vi "Halvorsen_MEMP_Fast.vi"(0 "tolerance":dbl=1e-13, 1 "Error Analysis":u16(ring)=4 items=["Max", "Max_Norm", "Norm", "Last Value", "Last Constant"], 3 "Шаг h, с":dbl=0.001, 4 "k":i32=4, 5 "Время, с":dbl=30.0, 7 "Hmax":dbl=0.5, 8 "Parameter":dbl[](array[numeric])=[1.4, 1.4, 1.4], 10 "last_point_Thomas":dbl[](array[numeric])=[2.3727475682665875, 0.23609824454436878, 0.4447912442126299], 13 "Hmin":dbl=0.001, 15 "Points count":i32=2, 18 "n":i32[](array[numeric])=[2, 4, 6, 8, 10, 12, 14, 16, 18, 20, 22], 19 "Ext.Type":u16(ring) items=["FNode", "MathScript", "ECD8 Arrays", "ECD8 Fnode", "ECD8 FnodeDiv", "FNode Exp"]) -> (6 "Elapsed Time":dbl=0.013410782656137599, 12 "Number of steps":i32=365, 14 "Error Estimation":dbl=1.511027811908779e-13, 17 "Rejected steps":i32=1)   [LabVIEW 2016]
uses:
  <vilib>/Analysis/_algsub.llb/Real Vector Norm.vi
  <vilib>/Analysis/5stat.llb/RMS (DBL).vi
  <vilib>/Analysis/NI_AALBase.lvlib
  <vilib>/Analysis/NI_AALPro.lvlib
panel:
  in  "Initial Conditions":dbl[](array[numeric])=[1.0, 0.0, 1.0]
  out "Last Value Reference":dbl[](array[numeric])=[2.372747575181197, 0.2360982473599586, 0.44479123807251236] format="%#_15f"
  out "Rejected Steps":i32[](graph)=[0, 1, 0, 0, 0, 0, 0, 0, 0, 0, 0, 0, 0, 0, 0, 0, 0, 0, 0, 0, 0, 0, 0, 0, 0, 0, 0, 0, 0, 0, 0, 0, 0, 0, 0, 0, 0, 0, 0, 0, 0, 0, 0, 0, 0, 0, 0, 0, 0, 0, 0, 0, 0, 0, 0, 0, 0, 0, 0, 0, 0, 0, 0, 0, 0, 0, 0, 0, 0, 0, 0, 0, 0, 0, 0, 0, 0, 0, 0, 0, 0, 0, 0, 0, 0, 0, 0, 0, 0, 0, 0, 0, 0, 0, 0, 0, 0, 0, 0, 0, 0, 0, 0, 0, 0, 0, 0, 0, 0, 0, 0, 0, 0, 0, 0, 0, 0, 0, 0, 0, 0, 0, 0, 0, 0, 0, 0, 0, 0, 0, 0, 0, 0, 0, 0, 0, 0, 0, 0, 0, 0, 0, 0, 0, 0, 0, 0, 0, 0, 0, 0, 0, 0, 0, 0, 0, 0, 0, 0, 0, 0, 0, 0, 0, 0, 0, 0, 0, 0, 0, 0, 0, 0, 0, 0, 0, 0, 0, 0, 0, 0, 0, 0, 0, 0, 0, 0, 0, 0, 0, 0, 0, 0, 0, 0, 0, 0, 0, 0, 0, 0, 0, 0, 0, 0, 0, 0, 0, 0, 0, 0, 0, 0, 0, 0, 0, 0, 0, 0, 0, 0, 0, 0, 0, 0, 0, 0, 0, 0, 0, 0, 0, 0, 0, 0, 0, 0, 0, 0, 0, 0, 0, 0, 0, 0, 0, 0, 0, 0, 0, 0, 0, 0, 0, 0, 0, 0, 0, 0, 0, 0, 0, 0, 0, 0, 0, 0, 0, 0, 0, 0, 0, 0, 0, 0, 0, 0, 0, 0, 0, 0, 0, 0, 0, 0, 0, 0, 0, 0, 0, 0, 0, 0, 0, 0, 0, 0, 0, 0, 0, 0, 0, 0, 0, 0, 0, 0, 0, 0, 0, 0, 0, 0, 0, 0, 0, 0, 0, 0, 0, 0, 0, 0, 0, 0, 0, 0, 0, 0, 0, 0, 0, 0, 0, 0, 0, 0, 0, 0, 0, 0, 0, 0, 0, 0, 0, 0, 0, 0, 0, 0, 0, 0, 0, 0, 0, 0, 0, 0, 0, 0, 0, 0, 0, 0, 0]
  out "Last Value":dbl[](array[numeric])=[2.372747568266689, 0.23609824454439432, 0.4447912442125211] format="%#_15f"
  out "Step time variation":dbl[](graph)=[0.011369601445039734, 0.015451963867235463]
  out "Real Error":dbl[][](graph)=[[0.0, 0.0, 0.0], [-3.3306690738754696e-16, 1.3010426069826053e-18, -2.220446049250313e-16], [2.269606724780715e-11, 7.413888947205294e-12, 4.742872761198669e-13], [4.520905871885361e-11, 1.3305856416678807e-11, 1.909139513145419e-12], [7.047429306794584e-11, 1.876210298235037e-11, 4.3729464493935666e-12], [9.8196561992836e-11, 2.377908980832899e-11, 8.00870481043603e-12], [1.2789103109867028e-10, 2.8306301746994222e-11, 1.2933210058463374e-11], [1.5886247872742842e-10, 3.224581712757413e-11, 1.921751646705161e-11], [1.901305779483664e-10, 3.5431102496374933e-11, 2.6864288571459838e-11], [2.2054869042165137e-10, 3.7660319307519785e-11, 3.5733416225980363e-11], [2.49152254383489e-10, 3.872691056727717e-11, 4.555289478958002e-11], [2.7525737245071014e-10, 3.842048901248063e-11, 5.593414620364001e-11], [2.9841329407531703e-10, 3.652400604181594e-11, 6.640399341506509e-11], [3.1840730052579147e-10, 3.281785954101224e-11, 7.643041755045488e-11], [3.351821042940628e-10, 2.706557200582438e-11, 8.546230390038545e-11], [3.488276334451257e-10, 1.9006352047767905e-11, 9.29043508790528e-11], [3.5940028730863105e-10, 8.411493723770036e-12, 9.811396139980388e-11], [3.670319603799044e-10, -4.916067553040193e-12, 1.003956917600135e-10], [3.719102803501073e-10, -2.1124657578752704e-11, 9.899281394609716e-11], [3.7423997234498074e-10, -4.012123966390391e-11, 9.306999615432687e-11], [3.7433145472220986e-10, -6.147837794401312e-11, 8.178391297519738e-11], [3.725815211907957e-10, -8.384315464127212e-11, 6.466382984626762e-11], [3.6960612348480026e-10, -1.0517831050549376e-10, 4.1951775386905865e-11], [3.6611647047379847e-10, -1.2337975086040842e-10, 1.4587886454364707e-11], [3.626872135953363e-10, -1.37165390157179e-10, -1.645572567099407e-11], [3.5965053157838156e-10, -1.458719811608944e-10, -5.041966844032686e-11], [3.571414275427287e-10, -1.493618562165011e-10, -8.721334765482425e-11], [3.5512126572712077e-10, -1.473818844743846e-10, -1.2639578272910512e-10], [3.535016723787976e-10, -1.398532400997965e-10, -1.6765255850259564e-10], [3.521241076498427e-10, -1.2682921379791878e-10, -2.1040236219960207e-10], [3.508104917671062e-10, -1.0861400667749876e-10, -2.537507981514864e-10], [3.493663136566738e-10, -8.573142196155459e-11, -2.969247070438996e-10], [3.4760949674250696e-10, -5.873412867174466e-11, -3.3953106992612447e-10], [3.453877184256271e-10, -2.8161695198036796e-11, -3.812243853928976e-10], [3.4256997238912845e-10, 5.6277205118249185e-12, -4.2203796013495776e-10], [3.3902347595926585e-10, 4.23832080542752e-11, -4.6196557690336704e-10], [3.346389831904162e-10, 8.190870204316525e-11, -5.009663794908192e-10], [3.2927260917858803e-10, 1.241433622567456e-10, -5.391123103493101e-10], [3.22812887532109e-10, 1.689934858717379e-10, -5.762417210064541e-10], [3.150950611541248e-10, 2.1638091318720853e-10, -6.122209406100865e-10], [3.0594549116358394e-10, 2.664068965430033e-10, -6.470637359257125e-10], [2.951319189037349e-10, 3.190443464973214e-10, -6.805551677757649e-10], [2.823865585810381e-10, 3.74259956359424e-10, -7.124398848645797e-10], [2.673807841802045e-10, 4.321243363136773e-10, -7.425686732176473e-10], [2.497113626986902e-10, 4.924811669582141e-10, -7.705183158179807e-10], [2.2885560113650172e-10, 5.552565074395943e-10, -7.960032633036462e-10], [2.0431967229228576e-10, 6.199005753160236e-10, -8.183853594800894e-10], [1.7554580011847065e-10, 6.856524237264239e-10, -8.370841797500361e-10], [1.421134321333284e-10, 7.512155342226379e-10, -8.514549065807842e-10], [1.0379430648299603e-10, 8.149392272116529e-10, -8.609801760428581e-10], [6.043654465770487e-11, 8.754437175184648e-10, -8.655169914106864e-10], [1.1836309710133719e-11, 9.318430471694228e-10, -8.651319660657464e-10], [-4.217692861629985e-11, 9.834488778892592e-10, -8.599161382960574e-10], [-1.0181278042864506e-10, 1.0298446539991346e-09, -8.499481118917629e-10], [-1.6732792929019524e-10, 1.070767030597608e-09, -8.352358804586402e-10], [-2.389262121482716e-10, 1.1059779758681998e-09, -8.157035047418049e-10], [-3.1656099963583983e-10, 1.1351612982934967e-09, -7.912341892790664e-10], [-4.003752884784717e-10, 1.1581864356458027e-09, -7.615919006553895e-10], [-4.902416250729402e-10, 1.1748908512743128e-09, -7.264904233750258e-10], [-5.856382045976716e-10, 1.1851151171526908e-09, -6.856295531321166e-10], [-6.8566397004588e-10, 1.1888712236896026e-09, -6.387324003043204e-10], [-7.88806797658026e-10, 1.1863856563820718e-09, -5.856388707314863e-10], [-8.927312222795081e-10, 1.1783156672606765e-09, -5.264999547449634e-10], [-9.954423951796798e-10, 1.1657244058937977e-09, -4.614766346833221e-10], [-1.095240786952445e-09, 1.1499659002822682e-09, -3.908151580134245e-10], [-1.1909015995570371e-09, 1.1324967630343963e-09, -3.1480018591878434e-10], [-1.282120631884709e-09, 1.1146310541221283e-09, -2.334257231950687e-10], [-1.3687890820790471e-09, 1.0976135556006739e-09, -1.4672596471143606e-10], [-1.4512280266387734e-09, 1.0825158547334013e-09, -5.4545479244438866e-11], [-1.5297518807244614e-09, 1.0703331554395845e-09, 4.319211655001709e-11], [-1.6049179762944732e-09, 1.0619474188899858e-09, 1.467421739675956e-10], [-1.6772010447141383e-09, 1.0581988618696414e-09, 2.5620083832222917e-10], [-1.7472245872340864e-09, 1.0598388833216177e-09, 3.718001462260645e-10], [-1.8155201786385078e-09, 1.0675997863529574e-09, 4.936342445915898e-10], [-1.8827255310327473e-09, 1.082119727158215e-09, 6.218509041033826e-10], [-1.9495254299783937e-09, 1.1040359737535255e-09, 7.567088067261807e-10], [-2.0165042968756097e-09, 1.1339031935619914e-09, 8.982441457305868e-10], [-2.0842634285145323e-09, 1.1722054438223495e-09, 1.0464090705042395e-09], [-2.153461409193369e-09, 1.219389034190499e-09, 1.20131138370283e-09], [-2.224737727374304e-09, 1.2758190059969365e-09, 1.3629377626500627e-09], [-2.298704337988511e-09, 1.3418079980453967e-09, 1.5312439094472552e-09], [-2.375939889276424e-09, 1.4175438600716461e-09, 1.706089047814885e-09], [-2.457072767469981e-09, 1.503223767684858e-09, 1.887440093106818e-09], [-2.542607457911572e-09, 1.5988392831900455e-09, 2.074995175682659e-09], [-2.633085305348004e-09, 1.7043637612346174e-09, 2.2685439082792414e-09], [-2.7290245618871722e-09, 1.8196844031592718e-09, 2.467889892443509e-09], [-2.8308635435791984e-09, 1.944516547780495e-09, 2.6726565405255087e-09], [-2.9390800904138814e-09, 2.0785546617219097e-09, 2.882632688105957e-09], [-3.0538354067743967e-09, 2.221035355631784e-09, 3.0969237174716113e-09], [-3.175532725663288e-09, 2.3713093710853173e-09, 3.315203667142441e-09], [-3.3041729352589755e-09, 2.5281736704130253e-09, 3.5363526551535074e-09], [-3.4395992720703816e-09, 2.690032196994707e-09, 3.7589874546384294e-09], [-3.581490215509575e-09, 2.8548599040334466e-09, 3.981411866860185e-09], [-3.729302644472909e-09, 3.020099725858927e-09, 4.201519576696455e-09], [-3.882181243142213e-09, 3.1824853863327007e-09, 4.41654868232888e-09], [-4.03904820700518e-09, 3.3380214148337473e-09, 4.62318183735988e-09], [-4.199012693106852e-09, 3.4821168171106365e-09, 4.8179054079611205e-09], [-4.36111946555684e-09, 3.608756848905159e-09, 4.995886815351014e-09], [-4.523064811579047e-09, 3.708372275923466e-09, 5.1477349050088606e-09], [-4.665753783328341e-09, 3.761142508551529e-09, 5.241526990218404e-09], [-4.778935247529148e-09, 3.7647316375455375e-09, 5.27045962428474e-09], [-4.867581893108763e-09, 3.7267104957550146e-09, 5.2449036225254986e-09], [-4.934693764724329e-09, 3.651821955941159e-09, 5.168978356451248e-09], [-4.982243506646e-09, 3.5434499778830286e-09, 5.043296669171582e-09], [-5.011369763607831e-09, 3.4055585018677448e-09, 4.867777292361097e-09], [-5.0233026627211075e-09, 3.2424267715214228e-09, 4.641494300017257e-09], [-5.019344051504504e-09, 3.0601361444837494e-09, 4.3650949521634175e-09], [-5.001047020947169e-09, 2.8651285788328096e-09, 4.0389944722107884e-09], [-4.970253653091561e-09, 2.6656907792244056e-09, 3.6668996727939884e-09], [-4.928755514832517e-09, 2.4691173550195344e-09, 3.250662405918092e-09], [-4.877563686278563e-09, 2.2806920796369923e-09, 2.784903418984186e-09], [-4.8176391764798154e-09, 2.1081003609424442e-09, 2.268234933211488e-09], [-4.749119153490966e-09, 1.9586847699315513e-09, 1.6932069080155543e-09], [-4.6732550607053724e-09, 1.8433663484529461e-09, 1.0728617994004708e-09], [-4.593981389744428e-09, 1.7714603117724437e-09, 4.6040993240126227e-10], [-4.512853715721299e-09, 1.7417605135960912e-09, -1.2046008635024918e-10], [-4.429691658619506e-09, 1.749222100499992e-09, -6.649663042423981e-10], [-4.344329868066765e-09, 1.787636705330442e-09, -1.1674967659303093e-09], [-4.256868690877269e-09, 1.849461916947348e-09, -1.622452394656193e-09], [-4.166818112771864e-09, 1.927224602127353e-09, -2.0314718796043962e-09], [-4.073079096222898e-09, 2.0147226109656913e-09, -2.40032660414613e-09], [-3.97467686541475e-09, 2.1065007516085643e-09, -2.733283821498844e-09], [-3.8703744653645344e-09, 2.198025761401823e-09, -3.0349061042045378e-09], [-3.759503153233368e-09, 2.2845947356131546e-09, -3.307053519918668e-09], [-3.6415166437819835e-09, 2.3617054978331e-09, -3.551469340834501e-09], [-3.515302271495102e-09, 2.4255042418985795e-09, -3.771099210680973e-09], [-3.3810777511078527e-09, 2.471259641367851e-09, -3.966069916927495e-09], [-3.2386722192967454e-09, 2.4946693599758873e-09, -4.137856501884585e-09], [-3.088418742969168e-09, 2.4911006590855322e-09, -4.287481480957922e-09], [-2.93190971500934e-09, 2.4558959310638784e-09, -4.415178667116493e-09], [-2.7711624106530053e-09, 2.3847972485668834e-09, -4.521777174915087e-09], [-2.608735893971925e-09, 2.2737820515317253e-09, -4.608395665073317e-09], [-2.4485620198078095e-09, 2.1201280731020233e-09, -4.676016907012581e-09], [-2.2952866274295047e-09, 1.922894732331315e-09, -4.725975166763874e-09], [-2.152907629948686e-09, 1.6809034164566583e-09, -4.760234872946967e-09], [-2.026153245182627e-09, 1.3948939781016634e-09, -4.780551510208397e-09], [-1.9199142275994063e-09, 1.0684315654430065e-09, -4.7886514753514575e-09], [-1.8381887123553042e-09, 7.05777658538409e-10, -4.786272822521198e-09], [-1.7843810873330312e-09, 3.1537883415921897e-10, -4.774996509304685e-09], [-1.7602175272912746e-09, -9.689493651876546e-11, -4.756135596473143e-09], [-1.766607971021017e-09, -5.262750235601743e-10, -4.73051503524502e-09], [-1.8039589821938762e-09, -9.692806557382028e-10, -4.698394673319228e-09], [-1.8729175987886038e-09, -1.4267333980910735e-09, -4.659212571311855e-09], [-1.9751693614011856e-09, -1.902701107781013e-09, -4.611367121487575e-09], [-2.112907848683676e-09, -2.39911290833561e-09, -4.55224062612114e-09], [-2.280200916970898e-09, -2.8884983294119593e-09, -4.480942660325948e-09], [-2.456705505693435e-09, -3.321690478230721e-09, -4.401077169369216e-09], [-2.632064344254559e-09, -3.7018246246134368e-09, -4.312903090220033e-09], [-2.8018853903688523e-09, -4.040882295441861e-09, -4.21502360792303e-09], [-2.9626983089059422e-09, -4.3464973842333166e-09, -4.105980500046513e-09], [-3.1108005060787036e-09, -4.622784821606274e-09, -3.984646002042069e-09], [-3.2425311324857375e-09, -4.87253881686911e-09, -3.85004728098437e-09], [-3.3539198085463795e-09, -5.0973394394304705e-09, -3.7016664178324277e-09], [-3.441230411738161e-09, -5.298790739516335e-09, -3.5389657870865676e-09], [-3.5004914522573927e-09, -5.4782338665404495e-09, -3.3616257555380002e-09], [-3.5272615939163643e-09, -5.636151101384712e-09, -3.1703967229290697e-09], [-3.5172265100413824e-09, -5.7729803160100346e-09, -2.966862755471311e-09], [-3.4662375192340278e-09, -5.889586596197205e-09, -2.7529919455204777e-09], [-3.3704501412046284e-09, -5.9867684143455335e-09, -2.5318758201109404e-09], [-3.2270670580203387e-09, -6.065342006422725e-09, -2.30813290702514e-09], [-3.034582807259767e-09, -6.126536611361644e-09, -2.0870680739193403e-09], [-2.7925790568872344e-09, -6.171990030168217e-09, -1.874124300194069e-09], [-2.5033464190471477e-09, -6.203366709200964e-09, -1.6756662724048965e-09], [-2.1715211850903415e-09, -6.222673043509985e-09, -1.4976326845328458e-09], [-1.8041537153123954e-09, -6.232016236396021e-09, -1.3450718316931898e-09], [-1.4073324727803538e-09, -6.233577209968644e-09, -1.2209957489517365e-09], [-9.88697568260477e-10, -6.2293068481267255e-09, -1.1275709255187394e-09], [-5.555640392174155e-10, -6.221014370311195e-09, -1.0656620030857766e-09], [-1.1039880121188617e-10, -6.210144842810905e-09, -1.0349947565657658e-09], [3.416795735233791e-10, -6.1979439358594846e-09, -1.0353415902386587e-09], [7.983995686799972e-10, -6.185412182446726e-09, -1.0661789229260421e-09], [1.2571450547227414e-09, -6.17340312203396e-09, -1.1269785105127994e-09], [1.7155787901401709e-09, -6.162597099290679e-09, -1.2171479379929906e-09], [2.1712422970665557e-09, -6.153543008480256e-09, -1.3359688910696832e-09], [2.622194905654851e-09, -6.146612108182126e-09, -1.4826724292760218e-09], [3.0670750383876566e-09, -6.1420393215882996e-09, -1.6565446792071725e-09], [3.50443807306533e-09, -6.139857955389516e-09, -1.8567787307688377e-09], [3.93260091158254e-09, -6.139864616727664e-09, -2.0823258672919565e-09], [4.3493675327965775e-09, -6.141575248364006e-09, -2.3316473196643983e-09], [4.752593429913077e-09, -6.144155406673235e-09, -2.602883242275311e-09], [5.139857428559935e-09, -6.146263498152393e-09, -2.893587813801446e-09], [5.507105438340432e-09, -6.145950859348659e-09, -3.199704945444637e-09], [5.847144546322625e-09, -6.140574271285004e-09, -3.513682456102174e-09], [6.151850584501517e-09, -6.126912754922387e-09, -3.825169070381662e-09], [6.414956121858495e-09, -6.101413152492796e-09, -4.123291486024527e-09], [6.631765803177814e-09, -6.0605684915060465e-09, -4.397124664379248e-09], [6.800017438024497e-09, -6.0011866587217355e-09, -4.637271011631583e-09], [6.919676831529387e-09, -5.920428147732082e-09, -4.836907985250605e-09], [6.991337953010657e-09, -5.816171100292422e-09, -4.99025554212551e-09], [7.016646819124617e-09, -5.686787929448656e-09, -5.093523824939439e-09], [6.997607382430715e-09, -5.5315445557369e-09, -5.143962145126579e-09], [6.93653423589069e-09, -5.34997135481774e-09, -5.14003661855611e-09], [6.835543020500268e-09, -5.141924219742577e-09, -5.080567078152853e-09], [6.695762388986282e-09, -4.906637540713632e-09, -4.96370322622397e-09], [6.517690831486789e-09, -4.643849527141697e-09, -4.786623541974677e-09], [6.3030773933547835e-09, -4.3561028117977685e-09, -4.547633380980187e-09], [6.062590429678494e-09, -4.0566199288605276e-09, -4.256597740948109e-09], [5.81213410733028e-09, -3.762749001268162e-09, -3.9333607482205935e-09], [5.556922699767597e-09, -3.4795997194692063e-09, -3.586301033919881e-09], [5.295042071473688e-09, -3.206297449764861e-09, -3.2140152761428453e-09], [5.029283212110158e-09, -2.9478257612680636e-09, -2.8218201109098118e-09], [4.780692619554827e-09, -2.7233629795730963e-09, -2.4437900592033657e-09], [4.5569121809307944e-09, -2.537292265181179e-09, -2.095620121878028e-09], [4.351461524443323e-09, -2.382397723543761e-09, -1.7708918775838356e-09], [4.159282807059128e-09, -2.2535548982460796e-09, -1.4644823131959583e-09], [3.97693200593352e-09, -2.147515165695779e-09, -1.1733036764383087e-09], [3.801982451090424e-09, -2.062131465585537e-09, -8.956360098011373e-10], [3.6326260888230877e-09, -1.9958757424554108e-09, -6.305684863150418e-10], [3.467354514619103e-09, -1.947516592437637e-09, -3.776414736478273e-10], [3.304651441382589e-09, -1.9159627218101605e-09, -1.3632250883688357e-10], [3.1432425551258802e-09, -1.9002852624794286e-09, 9.352696395126259e-11], [2.981949243086035e-09, -1.899621626666459e-09, 3.1190294791372253e-10], [2.81961448633794e-09, -1.9131453643517204e-09, 5.187579255050423e-10], [2.6553158005704347e-09, -1.940025556868008e-09, 7.137486157660078e-10], [2.487990868882406e-09, -1.9794431926900558e-09, 8.966849485148032e-10], [2.3167188167860786e-09, -2.0305581105439785e-09, 1.0671934447259446e-09], [2.1407650097060582e-09, -2.0924657007093117e-09, 1.2247727276815112e-09], [1.9593948685781015e-09, -2.164243492752682e-09, 1.3689147593254347e-09], [1.771992774735054e-09, -2.244921679106504e-09, 1.4990564345396251e-09], [1.5780284856603544e-09, -2.3334966979537963e-09, 1.6145866865713288e-09], [1.3771092044478905e-09, -2.428919117919426e-09, 1.7148815700807063e-09], [1.1690972911981845e-09, -2.5300416761631084e-09, 1.799220328280171e-09], [9.537731437969654e-10, -2.635785117943712e-09, 1.8669918944169694e-09], [7.312949135140911e-10, -2.744931448805943e-09, 1.9174906107366496e-09], [5.019145099538491e-10, -2.85626805540673e-09, 1.950104966397248e-09], [2.6597082869450617e-10, -2.968591344965077e-09, 1.9642665272101567e-09], [2.415462274640845e-11, -3.080595389892693e-09, 1.9595067790589837e-09], [-2.2280810529906603e-10, -3.1910176168103987e-09, 1.9354691183082195e-09], [-4.741609882508158e-10, -3.2986323117434324e-09, 1.8919426025831854e-09], [-7.289530090659468e-10, -3.4021760964009218e-09, 1.8288877079442045e-09], [-9.859847938109567e-10, -3.500330192363066e-09, 1.7464900636809944e-09], [-1.2443835961661875e-09, -3.591920649803626e-09, 1.6450409923152165e-09], [-1.502631796768128e-09, -3.6755704591051597e-09, 1.5253149854288495e-09], [-1.7599580681704197e-09, -3.7501592942135176e-09, 1.387996828583482e-09], [-2.015107303243724e-09, -3.814406901447853e-09, 1.2342380451002555e-09], [-2.26694063520938e-09, -3.867074993557651e-09, 1.0654308546520497e-09], [-2.5144488713380042e-09, -3.906978074397216e-09, 8.831460007741043e-10], [-2.756545547377698e-09, -3.93294807832234e-09, 6.893667858776098e-10], [-2.992597392115215e-09, -3.9439179699840565e-09, 4.859401769863325e-10], [-3.222195288365981e-09, -3.93883525795502e-09, 2.7474911235003674e-10], [-3.4446028251977623e-09, -3.916726609709542e-09, 5.8197446861640856e-11], [-3.659446079495865e-09, -3.876729604002094e-09, -1.6143797409995386e-10], [-3.866637454663646e-09, -3.818018678991564e-09, -3.8202063734615876e-10], [-4.065669245711945e-09, -3.7400819108412975e-09, -6.008025188464217e-10], [-4.256674901448321e-09, -3.6423702942656178e-09, -8.156786357460533e-10], [-4.439304923664622e-09, -3.5248239882434973e-09, -1.0239071812634393e-09], [-4.61362881232219e-09, -3.3873768234826684e-09, -1.2232712620630082e-09], [-4.778922813031272e-09, -3.2310505382326937e-09, -1.410646266464255e-09], [-4.93485519115211e-09, -3.0570281861486137e-09, -1.5835865951885353e-09], [-5.080536435997374e-09, -2.8677200614168896e-09, -1.7393224638340143e-09], [-5.214943810116779e-09, -2.6665073482590174e-09, -1.8754557906675018e-09], [-5.337447817055363e-09, -2.4566448875162905e-09, -1.990664966200484e-09], [-5.447135853486884e-09, -2.2423392032067113e-09, -2.083982764133907e-09], [-5.54339196767728e-09, -2.027551238015235e-09, -2.1554211748764374e-09], [-5.625971466471924e-09, -1.8153105685314586e-09, -2.205847504654912e-09], [-5.694684057644395e-09, -1.6084760190437919e-09, -2.236585583403894e-09], [-5.7495230798565444e-09, -1.409225736104247e-09, -2.2493913398591303e-09], [-5.790611989908712e-09, -1.2192902243413073e-09, -2.24628271539018e-09], [-5.818211690211683e-09, -1.0395844185495662e-09, -2.22945928385343e-09], [-5.83263015663249e-09, -8.708156418180124e-10, -2.201194337914103e-09], [-5.834265959236973e-09, -7.133907353740199e-10, -2.163833556778627e-09], [-5.823457049913827e-09, -5.670461877826938e-10, -2.1196204791351647e-09], [-5.80073256095659e-09, -4.319352098214324e-10, -2.0709585157874244e-09], [-5.766574773247157e-09, -3.0767166592227113e-10, -2.020194234120254e-09], [-5.7215274740229916e-09, -1.9384145677481257e-10, -1.9696750896969206e-09], [-5.666408675608636e-09, -9.015454355276731e-11, -1.9218662217213023e-09], [-5.601418884282339e-09, 4.390068170101458e-12, -1.8789343414482573e-09], [-5.527749147304917e-09, 8.995805489409037e-11, -1.8434294091207448e-09], [-5.4457218734427215e-09, 1.6742940367464598e-10, -1.8175621008253984e-09], [-5.356866061845267e-09, 2.36987263146915e-10, -1.8037153992622734e-09], [-5.261604263395725e-09, 2.9939045687044086e-10, -1.8039747473608259e-09], [-5.1615165475027425e-09, 3.5483671556590934e-10, -1.8202950258228157e-09], [-5.057974927780151e-09, 4.0360109698767133e-10, -1.854307818405232e-09], [-4.9523753986591146e-09, 4.458652336225555e-10, -1.9072334822567427e-09], [-4.846209211706309e-09, 4.816845811106418e-10, -1.9798287453909325e-09], [-4.741064651980764e-09, 5.110044609679676e-10, -2.0723378568732187e-09], [-4.638801787137936e-09, 5.336596720084685e-10, -2.184266989502248e-09], [-4.540727349677809e-09, 5.495457422455274e-10, -2.314815894521871e-09], [-4.448753809782602e-09, 5.585499840421448e-10, -2.4622490712999934e-09], [-4.3638210822649626e-09, 5.607743158719813e-10, -2.624872763590247e-09], [-4.286983545931378e-09, 5.565270466689753e-10, -2.800431886385013e-09], [-4.218372651187963e-09, 5.463909324987526e-10, -2.9869964279782835e-09], [-4.157505228974401e-09, 5.311366901850079e-10, -3.1830156288492617e-09], [-4.103854700510112e-09, 5.117533063980773e-10, -3.3868703397388344e-09], [-4.056622593395787e-09, 4.894056271353975e-10, -3.597298459112608e-09], [-4.015071664031922e-09, 4.6547588006262686e-10, -3.813056537183002e-09], [-3.978497309375939e-09, 4.4156212020141083e-10, -4.032954414867618e-09], [-3.946223126050086e-09, 4.194657954315062e-10, -4.2559422652743706e-09], [-3.917713709000736e-09, 4.0122904998440845e-10, -4.480912529913894e-09], [-3.892517780323956e-09, 3.890865407640831e-10, -4.7068784425619015e-09], [-3.870330403388245e-09, 3.8546854597143465e-10, -4.93293050851662e-09], [-3.85102752117894e-09, 3.92987642428011e-10, -5.158182325715188e-09], [-3.834685985415476e-09, 4.144173892939307e-10, -5.381816770011483e-09], [-3.821613053789363e-09, 4.526679031613412e-10, -5.6031286277402614e-09], [-3.812387822099694e-09, 5.107811951177155e-10, -5.821636506198047e-09], [-3.807897219765266e-09, 5.918958656536688e-10, -6.0369211851707405e-09], [-3.8092679566226195e-09, 6.987410650083348e-10, -6.247987904828278e-09], [-3.8179840400331955e-09, 8.341660695521114e-10, -6.454676793055114e-09], [-3.835707973465219e-09, 1.0002243477913453e-09, -6.656261319903933e-09], [-3.8642820054946014e-09, 1.1983645187285674e-09, -6.852263645384937e-09], [-3.90582499676384e-09, 1.4299228467962166e-09, -7.0428507470410295e-09], [-3.962628891684972e-09, 1.6958523474386311e-09, -7.228353915422758e-09], [-4.036962431008817e-09, 1.9962462793898794e-09, -7.409041380412873e-09], [-4.1313410470422696e-09, 2.3314044028666103e-09, -7.585816419464209e-09], [-4.247999951800807e-09, 2.700488277440627e-09, -7.759210607360956e-09], [-4.389414720584739e-09, 3.103089785128077e-09, -7.93030396906147e-09], [-4.557411115158061e-09, 3.5373051154863333e-09, -8.099655168791742e-09], [-4.75349570816519e-09, 4.0008458768170385e-09, -8.26786283880665e-09], [-4.9787550748803255e-09, 4.491029770292698e-09, -8.435508291881888e-09], [-5.233573685536896e-09, 5.0045096955386725e-09, -8.602911716337758e-09], [-5.5185711556049455e-09, 5.538823621975553e-09, -8.770680626213334e-09], [-5.833511340647135e-09, 6.090664417257585e-09, -8.938944695557893e-09], [-6.177853562050473e-09, 6.656840856322788e-09, -9.107663956342549e-09], [-6.550929798621041e-09, 7.234412624512743e-09, -9.276642565225757e-09], [-6.951584641257114e-09, 7.82024223155986e-09, -9.445252580064789e-09], [-7.377040533995682e-09, 8.40979508254236e-09, -9.611983209367736e-09], [-7.825429637620118e-09, 9.000035827710917e-09, -9.775360076957895e-09], [-8.292970976597758e-09, 9.586286875418182e-09, -9.932703548543032e-09], [-8.773659132543798e-09, 1.016230699590892e-08, -1.0080096313203057e-08], [-9.258922739618924e-09, 1.0720217158421974e-08, -1.0212181322799552e-08], [-9.7368848539503e-09, 1.1250214981828321e-08, -1.032212937346344e-08], [-1.0191253840829972e-08, 1.1739953009737292e-08, -1.0401828731687601e-08], [-1.0604467970409814e-08, 1.2177236996535612e-08, -1.0443685916072809e-08], [-1.096367463482295e-08, 1.255452142245872e-08, -1.0442121389786507e-08], [-1.1259140064723283e-08, 1.2867233278868184e-08, -1.0393014004961287e-08], [-1.148353523383605e-08, 1.3113111041462844e-08, -1.0293208063671955e-08], [-1.1630587604116727e-08, 1.3290921030417735e-08, -1.014061479231998e-08], [-1.1695501678232745e-08, 1.340079092138069e-08, -9.934014499890509e-09], [-1.1674525346450082e-08, 1.3443786084366138e-08, -9.673084555572586e-09], [-1.156482420938687e-08, 1.342175859342376e-08, -9.358395391956265e-09], [-1.1363736396319268e-08, 1.3336967752408668e-08, -8.990389765983764e-09], [-1.1068054028839924e-08, 1.3191571168746918e-08, -8.569500442590083e-09], [-1.0673199213329099e-08, 1.2987354303106713e-08, -8.095681902631213e-09], [-1.017599293717808e-08, 1.2727391363043239e-08, -7.57226303882419e-09], [-9.588436267193856e-09, 1.2423363004998578e-08, -7.019104408811927e-09], [-8.93945939495211e-09, 1.2095057844163648e-08, -6.468044100316206e-09], [-8.245271132523158e-09, 1.1754038520273014e-08, -5.932959901144841e-09], [-7.511117505742959e-09, 1.140538818944492e-08, -5.418163029347056e-09], [-6.7426513261636956e-09, 1.1053686410633645e-08, -4.929623598215471e-09], [-5.955683057834449e-09, 1.0706950881456123e-08, -4.479883131125462e-09], [-5.174996875467741e-09, 1.0375102110771195e-08, -4.0832999204099e-09], [-4.4158872114508085e-09, 1.0062462640902936e-08, -3.744493826118855e-09], [-3.681811300282334e-09, 9.768004016752485e-09, -3.460716602177172e-09], [-2.9716384908340387e-09, 9.488854091355137e-09, -3.22770010718898e-09], [-2.2837300939215766e-09, 9.221992836039306e-09, -3.0417879326449793e-09], [-1.616940359383534e-09, 8.964612996376076e-09, -2.9000659651501337e-09], [-9.703096104374254e-10, 8.713974597451823e-09, -2.800072285147337e-09], [-3.4311442576040463e-10, 8.46740752513675e-09, -2.7396788171429876e-09], [2.6449997747590714e-10, 8.222548170122579e-09, -2.7170038441326483e-09], [8.528102668492465e-10, 7.976860588732038e-09, -2.730222992131104e-09], [1.4215109089832367e-09, 7.728032824783071e-09, -2.7775797217799436e-09], [1.9701253961557086e-09, 7.473840130112208e-09, -2.8573112209606677e-09], [2.498349527257915e-09, 7.212025518454901e-09, -2.967699391787093e-09], [3.005254267662849e-09, 6.940663835330874e-09, -3.106926105278518e-09], [3.490032707276214e-09, 6.657897178019567e-09, -3.2731764104676486e-09], [3.9519369998686216e-09, 6.361928081566326e-09, -3.4647139844634633e-09], [4.3896632995199525e-09, 6.051398340756187e-09, -3.679645345366911e-09], [4.801834041501252e-09, 5.725244334175983e-09, -3.916026544703577e-09], [5.187472229550849e-09, 5.382309722912204e-09, -4.172227896503955e-09], [5.544876113816599e-09, 5.022221860606635e-09, -4.4462772352815705e-09], [5.872742292467592e-09, 4.644586076851809e-09, -4.736539105376636e-09], [6.1695231146075e-09, 4.249559037994288e-09, -5.041283890339088e-09], [6.4338507854699856e-09, 3.837423767638626e-09, -5.359055310627525e-09], [6.664240270737309e-09, 3.4090899825311993e-09, -5.688276183413166e-09], [6.859551593407787e-09, 2.965453077541369e-09, -6.027773225003585e-09], [6.914507633126732e-09, 2.815564281721805e-09, -6.14000872367626e-09]]
  out "Step Variation":dbl[](graph)=[0.001, 0.5, 0.07823061881315105, 0.07933192271624835, 0.08040574395300924, 0.0814016864180507, 0.0822729393920006, 0.08289550160111961, 0.08320062610554346, 0.08328219136937605, 0.08327785477235997, 0.08327533303798279, 0.08339913366608054, 0.08375034866855918, 0.08445094967473141, 0.0854452993812646, 0.08681096609432988, 0.08859409646886221, 0.09066485431127756, 0.0929238375980842, 0.09467387035462635, 0.0955119460900902, 0.09530922549851537, 0.09467462489661788, 0.09394521423176183, 0.09376677722185356, 0.09364675139677955, 0.09362821116763087, 0.09343866341894287, 0.09278593187833566, 0.09173955823965829, 0.09060880864926628, 0.08939086593124711, 0.08842432802759628, 0.08765939507068238, 0.08709162712896647, 0.08682558283775986, 0.086661337752421, 0.08659353718208354, 0.08687489696382773, 0.08724093269704253, 0.08769161220558877, 0.08839375472588404, 0.08907570632683971, 0.08992926392268197, 0.09052524197069017, 0.0908488356759059, 0.09059976065188788, 0.08962992344512015, 0.08827296408764118, 0.08692598031785441, 0.08567002994501932, 0.0846937430652111, 0.0840641473518584, 0.08377070729089624, 0.0836426663621795, 0.08390122532091562, 0.08438881250546795, 0.08496601656278864, 0.08551498705187167, 0.08580406457778471, 0.08547413053392132, 0.08471408445119624, 0.08356620134242214, 0.08212101650734498, 0.08075383534372005, 0.07943173580206102, 0.07831542203244932, 0.07731532458663018, 0.07655159781953236, 0.07588950557095803, 0.07540999326388587, 0.07501683891573553, 0.0747437050832594, 0.07463812052171052, 0.07458396856582769, 0.07455492531863607, 0.07462872721218437, 0.07475785756469744, 0.07494076134696222, 0.07515157716808732, 0.07544759530131377, 0.07575144637597699, 0.0761200722179067, 0.07658185613939361, 0.07711357063538096, 0.07780527793036501, 0.07851002695698361, 0.07945989953003683, 0.0805133507278289, 0.0817090480997369, 0.0831023314982851, 0.08475961626801558, 0.08674003598466369, 0.08921792173388177, 0.09264740815381747, 0.09753225060246253, 0.10398437859906483, 0.10281589097663144, 0.09613758598333602, 0.09217425657931147, 0.0900739786751866, 0.08946197350867678, 0.08948827037075503, 0.09020719815708461, 0.0910872973710579, 0.09231561384793206, 0.09336971731991808, 0.09475611270011694, 0.09751326418878155, 0.10088816299540816, 0.10560693583804544, 0.10934954898937788, 0.10818195373300667, 0.10525180932425135, 0.10236126913360061, 0.09915556025705481, 0.09530631662078327, 0.0915799509253442, 0.0886231917388381, 0.08628874312738186, 0.0847699343661121, 0.08360584266838418, 0.08279785554537021, 0.0827837544922971, 0.08282046327592936, 0.08333950217672648, 0.08425455619267037, 0.08517302165404754, 0.08621362698325635, 0.08744515238957253, 0.08850458207827046, 0.08926326972986644, 0.09024237580998352, 0.09113006463761922, 0.09162802105056686, 0.09192569121197314, 0.09153257715612466, 0.09105599587762778, 0.09069633490757248, 0.0906283876310104, 0.09144161783465386, 0.0935486952074855, 0.09668311272360017, 0.09705766206348825, 0.09119248906984226, 0.08546739976471109, 0.08142997049168652, 0.07867121216589136, 0.07671484318457916, 0.07538924977257173, 0.0744724426723474, 0.07404417854194936, 0.07408629168987227, 0.07433345379239988, 0.07471729514606701, 0.07534111499812399, 0.07608823809925946, 0.07673517792099549, 0.0772680834959627, 0.07776541976092702, 0.07792761590077844, 0.07769292301496773, 0.0769761390338545, 0.07612778779173346, 0.07499195752980843, 0.07364904486257046, 0.07268631715970095, 0.07169155884774796, 0.07096688307562436, 0.07041724614399289, 0.07003723443217723, 0.0697848605675002, 0.06970476890867663, 0.06985971361254341, 0.07024941465416283, 0.07086302239369255, 0.07167067137439888, 0.07273416080264508, 0.07409253121604124, 0.07560884462142885, 0.07685335328907233, 0.07758206385519936, 0.07790632550473972, 0.07784003559360335, 0.07754903225525889, 0.07737595742717285, 0.07724526468074948, 0.07738792620387028, 0.07774512541692158, 0.0785573930091561, 0.07995326721334113, 0.08233682985152747, 0.08573377620051771, 0.08970214215631284, 0.09186122428665369, 0.09134922529740376, 0.09125400261554865, 0.0932472459888935, 0.09566287386869854, 0.09249214758351651, 0.0867108272574912, 0.08260790709781236, 0.07989376419567255, 0.07810137427703663, 0.07690014574396958, 0.07606936779632904, 0.0754943715922761, 0.07518812822350962, 0.07505320907250826, 0.07505102932607093, 0.07518080451312299, 0.0753487210192737, 0.0756277638723026, 0.07597333375352897, 0.07632922530771258, 0.0767235735010964, 0.07714082942586026, 0.07758295215016407, 0.07803885567412547, 0.0784600083903329, 0.07892428796153061, 0.07934727691745412, 0.07975054524546155, 0.08015424297573183, 0.0804940328372191, 0.0808048547839219, 0.08111821614564882, 0.08140774861428711, 0.08162695116722646, 0.08189691053110343, 0.08203506761468514, 0.0822751128601768, 0.08246820985701209, 0.0826398246573662, 0.08281472304306055, 0.08294052515744045, 0.08314055039718113, 0.08346843000734201, 0.08377859237753373, 0.08416702413056261, 0.08472550555874597, 0.08525860485397674, 0.086019654713006, 0.08679417429724513, 0.08778375267826383, 0.08861084372234736, 0.08946739890993942, 0.09006144209363416, 0.0902599762370685, 0.09028542957052123, 0.08988227891287061, 0.08915120651648349, 0.08834437735084692, 0.0874080781546836, 0.08643665622514242, 0.08543952731569125, 0.08457806537529308, 0.08380137188344144, 0.08310595381722889, 0.08269701299980506, 0.08228602341740886, 0.08205342221368592, 0.08195583147297936, 0.08184132578373948, 0.0821674592504128, 0.08231231669481293, 0.08283040007330297, 0.08311640735829061, 0.08377129610514494, 0.08427899635646487, 0.08478756773419882, 0.08531100347269135, 0.08582137400271254, 0.08627387050273831, 0.0865060534120977, 0.08668754154650178, 0.08638800203056711, 0.08588874292476875, 0.08486200066717374, 0.08358566169446205, 0.0823267704715385, 0.08100343360723106, 0.07983189366100987, 0.07875377663488366, 0.07778658568188752, 0.07699499874410488, 0.07627944374211934, 0.07570697460067209, 0.07528839300332509, 0.07499036576398695, 0.07480201785233247, 0.07474184499830229, 0.0748556869039852, 0.07511853495809494, 0.07519640959188029, 0.07540719645697393, 0.07541728178880945, 0.07523805310433546, 0.07507139800891828, 0.0749247256019655, 0.07468677815524924, 0.07456106061699226, 0.07435291925120975, 0.07428659817082864, 0.07410502399758387, 0.07385513678429642, 0.07355748884118257, 0.07317315016440627, 0.07292761184330182, 0.0727186618999792, 0.07261526770874391, 0.07271002942516452, 0.07302683287510621, 0.07341974666707056, 0.07422644057819569, 0.07532491870855398, 0.07662634962140163, 0.07803500530177267, 0.07934241913117038, 0.0799997348851061, 0.07966584332602365, 0.07894199970120272, 0.07815735303034033, 0.0776095590452625, 0.07723832759710267, 0.07717305956608395, 0.07744553639568598, 0.07809409124720038, 0.07937535561690334, 0.08143930656415374, 0.08454030354588705, 0.08831758287822791, 0.09037767042025442, 0.08922930089433716, 0.08792640227894148, 0.08778911461063224, 0.08835249335457396, 0.08815107487323998, 0.08607910706870602, 0.08319025869959429, 0.08062535931129172, 0.07868519497757617, 0.07728063775801602, 0.0762666361400608, 0.07556925514438732, 0.07513134480177576, 0.07482743012762424, 0.07470131088302774, 0.0746753418557643, 0.0747294601758675, 0.07489104893239418, 0.07508409284904911, 0.07532860059428642, 0.07565150452349605, 0.07598325652294526, 0.07631169103405093, 0.07672623204772774, 0.07710369232169666, 0.07752547953372409, 0.07793993119008882, 0.07839109236133344, 0.07881886830416002, 0.07929068815144615, 0.025848048211901897, 0.0]
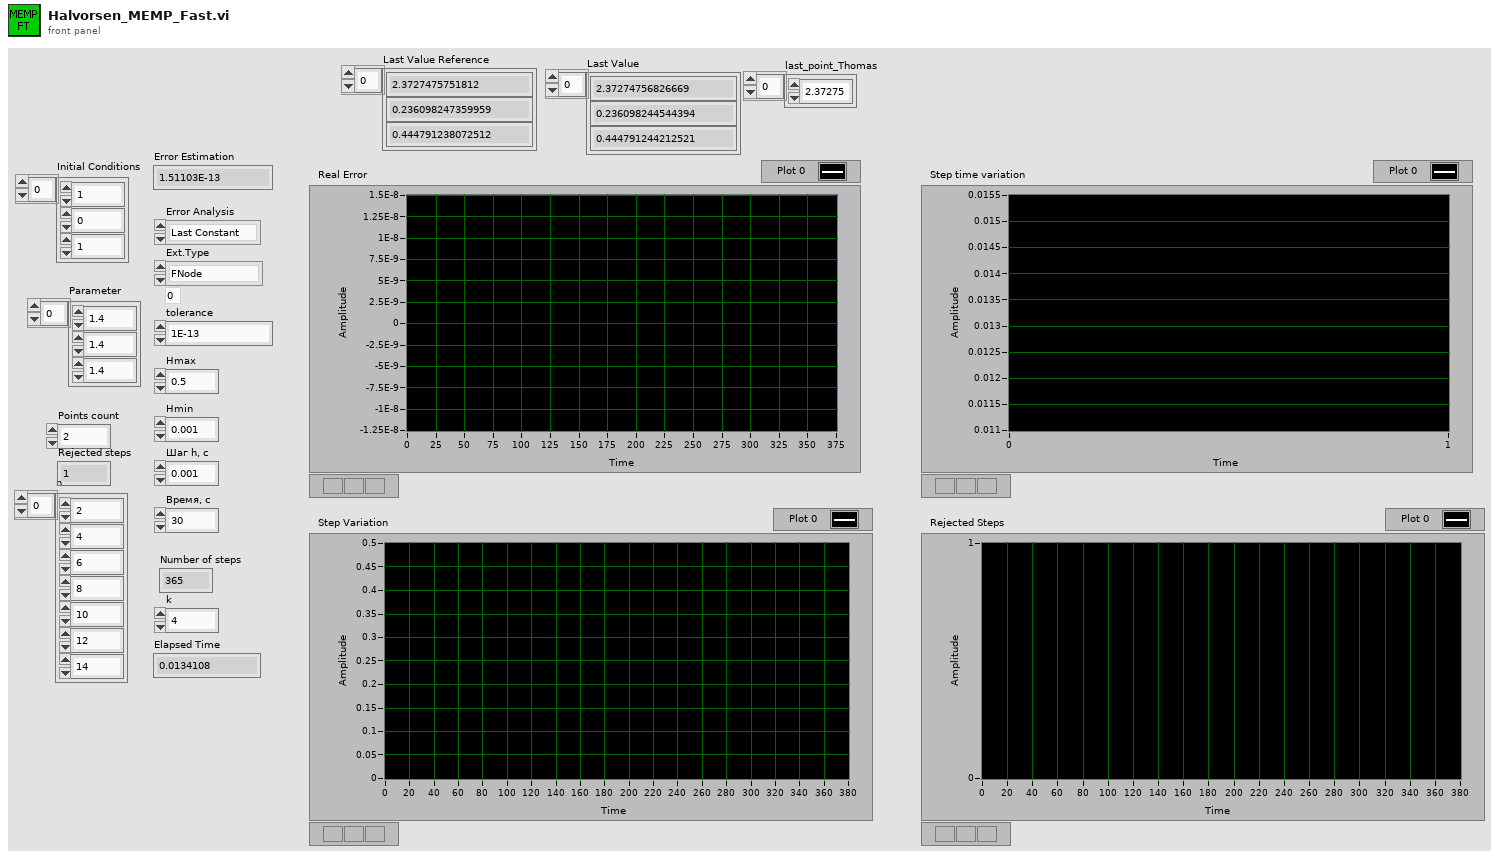
[diagram p1: front panel]
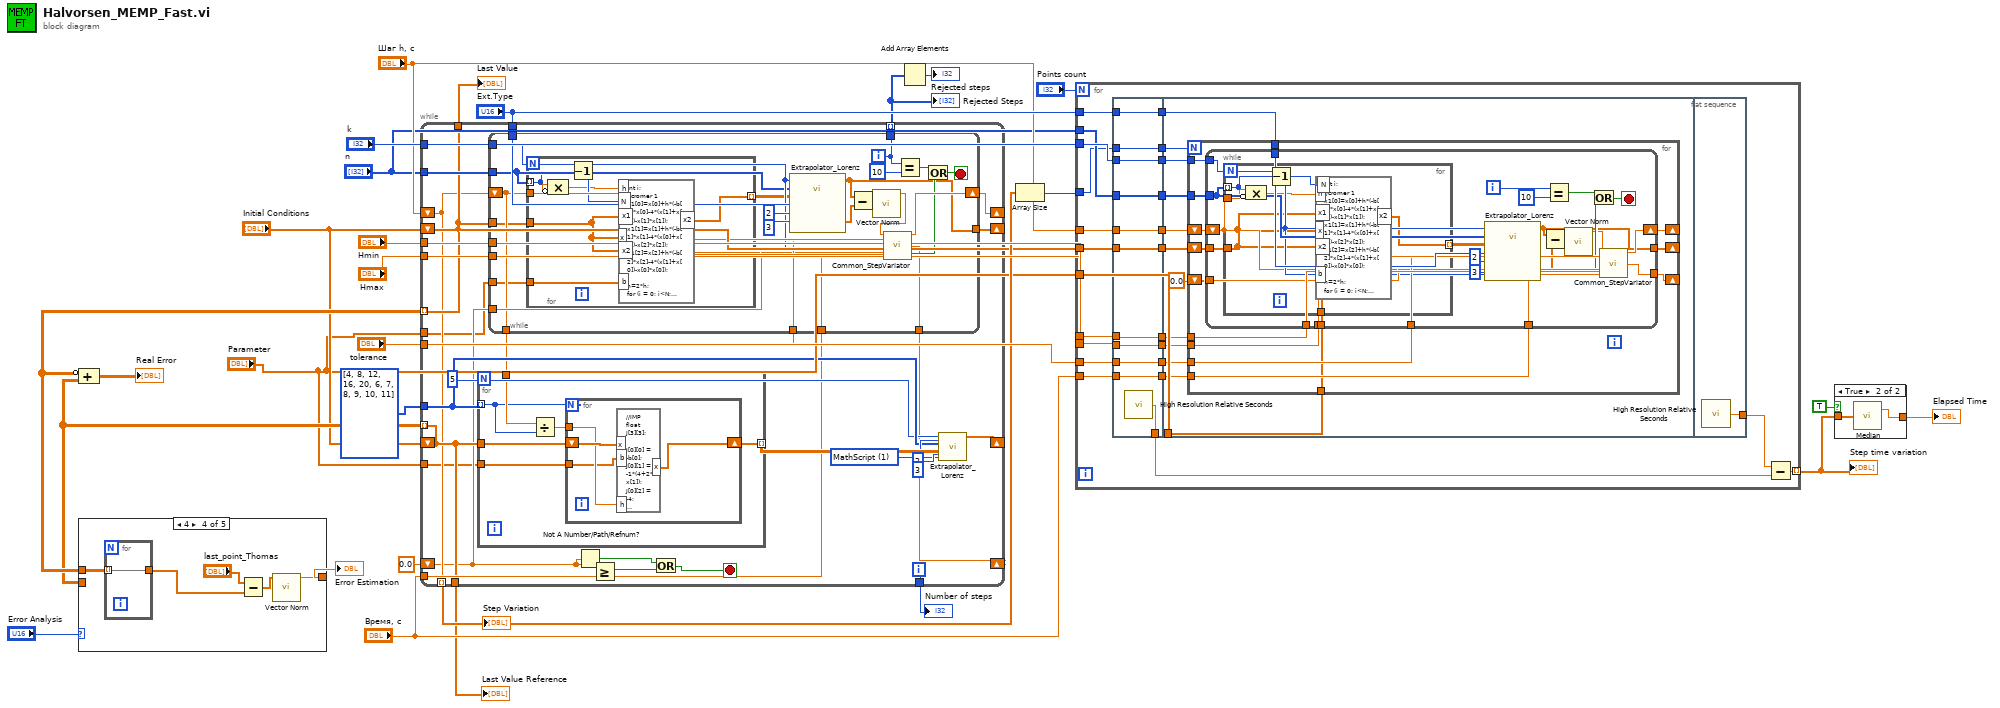
[diagram p0: block diagram]
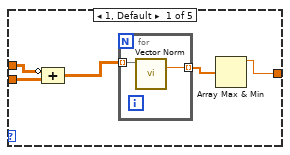
[diagram p2: hidden frame]
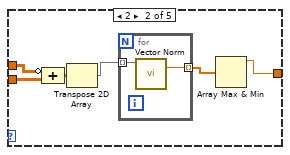
[diagram p3: hidden frame]
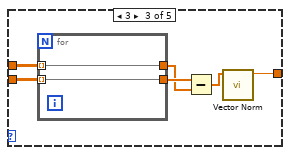
[diagram p4: hidden frame]
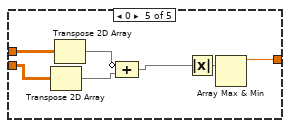
[diagram p5: hidden frame]
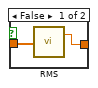
[diagram p6: hidden frame]
diagram:
  n1 = while {
    shift-right: [w50] -> _
    shift-left: "Initial Conditions" -> [w40]
    tunnel: "n" -> [w57]
    tunnel: "k" -> [w55]
    tunnel: "Ext.Type" -> [w45]
    shift-right: [w54] -> _
    shift-left: "Шаг h, с" -> [w35]
    shift-right: [w42] -> _
    shift-left: 0.0 -> [w31]
    tunnel: [w35] -> w13 mode=indexing
    tunnel: "Время, с" -> [w41]
    tunnel: [w56] -> w23
    tunnel: "tolerance" -> [w51]
    tunnel: "Hmin" -> [w53]
    tunnel: "Hmax" -> [w52]
    tunnel: [w40] -> w6 mode=indexing
    shift-right: [w49] -> _
    shift-left: "Initial Conditions" -> [w37]
    tunnel: i32[] [4, 8, 12, 16, 20, 6, 7, 8, 9, 10, 11] ("n 2") -> [w44]
    tunnel: [w37] -> w5 mode=indexing
    tunnel: [w40] -> w11
    tunnel: [w38] -> w10 mode=indexing
    tunnel: [w37] -> w4
    tunnel: "Parameter" -> [w30]
    tunnel: "Parameter" -> [w29]
    i -> [w56]
    stop <- w32 stop-if-true
    w36 = u16 1 items=["FNode", "MathScript", "ECD8 Arrays", "ECD8 Fnode", "ECD8 FnodeDiv"] ("Ext.Type")
    w43 = 5
    n2 = while {
      tunnel: w57 -> [w66]
      tunnel: w55 -> [w67]
      tunnel: w53 -> [w81]
      tunnel: w52 -> [w80]
      tunnel: w51 -> [w79]
      tunnel: [w60] -> w50
      tunnel: w45 -> [w76]
      tunnel: [w69] -> w42
      tunnel: w41 -> [w75]
      tunnel: w40 -> [w64]
      shift-right: [w82] -> w54
      shift-left: w35 -> [w65]
      tunnel: [w65] -> w39
      tunnel: [w70] -> w38
      tunnel: w31 -> [w68]
      tunnel: w30 -> [w62]
      i -> [w70]
      stop <- w72 stop-if-true
      n3 = for {
        N: w67 -> [_]
        tunnel: w66 -> [w88] mode=indexing
        tunnel: w65 -> [w89]
        tunnel: w64 -> [w87]
        tunnel: [w84] -> w63 mode=indexing
        tunnel: w62 -> [w83]
        n4 = Compound Arithmetic op=MULTIPLY(w89, invert w88) -> (w85:dbl)
        n5 = Decrement(x=w88) -> (x-1=w86:i32)
        n6 = formula code="int i;\n//cromer 1\nx1[0]=x[0]+h*(-b[0]*x[0]-4*(x[1]+x[2])-x[1]*x[1]);\nx1[1]=x[1]+h*(-b[1]*x[1]-4*(x[0]+x[2])-x[2]*x[2]);\nx1[2]=x[2]+h*(-b[2]*x[2]-4*(x[1]+x[0])-x[0]*x[0]);\n\nh=2*h;\nfor (i = 0; i<N; i++)\n{\n//EEuler\nx2[0]=x[0]+h*(-b[0]*x1[0]-4*(x1[1]+x1[2])-x1[1]*x1[1]);\nx2[1]=x[1]+h*(-b[1]*x1[1]-4*(x1[0]+x1[2])-x1[2]*x1[2]);\nx2[2]=x[2]+h*(-b[2]*x1[2]-4*(x1[1]+x1[0])-x1[0]*x1[0]);\n\nx[0]=x1[0];\nx[1]=x1[1];\nx[2]=x1[2];\nx1[0]=x2[0];\nx1[1]=x2[1];\nx1[2]=x2[2];\n};\n\nh=h*0.5;\nx2[0]=(x[0]+x1[0]+h*(-b[0]*x1[0]-4*(x1[1]+x1[2])-x1[1]*x1[1]))/2;\nx2[1]=(x[1]+x1[1]+h*(-b[1]*x1[1]-4*(x1[0]+x1[2])-x1[2]*x1[2]))/2;\nx2[2]=(x[2]+x1[2]+h*(-b[2]*x1[2]-4*(x1[1]+x1[0])-x1[0]*x1[0]))/2;"("x"=w87, "x1"=w87, "h"=w85, "x2"=w87, "N"=w86, "b"=w83) -> ("x2"=w84:dbl[])
      }
      n7 = call "Extrapolator_Lorenz.vi"("Порядок экстраполятора"=2 ("input variable"), "Dimension"=3 ("input variable"), "Ext.Type"=w76, "Х - нач. условия"=w63, "n"=w66, "k"=w67) -> ("TPrev"=w59:dbl[], "Tout"=w60:dbl[])  [unwired: 4 in]
      n8 = Subtract(x=w60, y=w59) -> (x-y=w61:dbl[])
      n9 = call-poly <vilib>:"Vector Norm.vi"("Input Vector"=w61) -> ("norm"=w58:dbl)  [unwired: 9 in, 1 out]
      n10 = call "Common_StepVariator.vi"("err"=w58, "tolerance"=w79, "Hmax"=w80, "Шаг h, с"=w65, "Current time"=w68, "k"=w67, "Hmin"=w81, "tmax"=w75) -> ("Hnew"=w82:dbl, "New time"=w69:dbl, "stop"=w71:bool)  [unwired: 4 in, 1 out]
      n11 = Equal?(x=w70, y=10) -> (x = y?=w74:bool)
      n12 = Or(x=w74, y=w71) -> (x .or. y?=w72:bool)
    }
    n13 = for {
      N: w43 -> [_]
      tunnel: w44 -> [w92] mode=indexing
      tunnel: w39 -> [w95]
      tunnel: w37 -> [w94]
      tunnel: [w91] -> w48 mode=indexing
      tunnel: w29 -> [w90]
      n14 = Divide(x=w95, y=w92) -> (x/y=w93:dbl)
      n15 = for {
        N: w92 -> [_]
        tunnel: w93 -> [w97]
        shift-right: [w99] -> w91
        shift-left: w94 -> [w98]
        tunnel: w90 -> [w96]
        n16 = formula code="//IMP\nfloat J[3][3];\n\nJ[0][0] = -b[0]; \nJ[0][1] = -1*(4+2*x[1]); \nJ[0][2] = -4; \n\nJ[1][0] = -4; \nJ[1][1] = -b[1];\nJ[1][2] = -1*(4+2*x[2]);\n\nJ[2][0] = -1*(4+2*x[0]); \nJ[2][1] = -4;\nJ[2][2] = -b[2];\n\n\nfloat w[3][4], Z[3], a[3], Zn[3], dz;\nfloat tol;\nint k; int i; int j; float t; float d;\ntol = 1e-14;\nint nnewtmax = 3, nnewt;\ndz = 2e-13;\nnnewt = 0;\n\nZ[0] = x[0]; Z[1] = x[1]; Z[2] = x[2];\nwhile ( (dz > tol) && (nnewt < nnewtmax)){\n\tfor(i=0;i<3;i++)\n\t{\n\t\tfor(j=0;j<3;j++)\n\t\t{\n\t\t\tif (i==j)\n\t\t\tw[i][j]=1 - 0.5*h*J[i][j];\n\t\t\telse\n\t\t\tw[i][j]= - 0.5*h*J[i][j];\n\t\t}\n\t}\n\n\n\n\ta[0] = 0.5*(x[0] + Z[0]);\n\ta[1] = 0.5*(x[1] + Z[1]);\n\ta[2] = 0.5*(x[2] + Z[2]);\n\t\n\tw[0][3]= -Z[0]+x[0]+h*(-b[0]*a[0]-4*(a[1]+a[2])-a[1]*a[1]);\n\tw[1][3]= -Z[1]+x[1]+h*(-b[1]*a[1]-4*(a[0]+a[2])-a[2]*a[2]);\n\tw[2][3]= -Z[2]+x[2]+h*(-b[2]*a[2]-4*(a[1]+a[0])-a[0]*a[0]);\n\t\n\t\n\tfor(k = 0; k <= 1; k++){\n\t\tint l = k;\n\t\n\t\tfor( i = k+1; i<= 2; i++){\n\t\t\tif( abs(w[i][k]) > abs(w[l][k]) ){\n\t\t\tl = i;\n\t\t\t}\n\t\t}\n\t\tif (l != k){\n\t\t\tfor( j = 0; j <= 3; j++){\n\t\t\t\tif ((j == 0) || (j >= k)){\n\t\t\t\t\tt = w[k][j];\n\t\t\t\t\tw[k][j] = w[l][j];\n\t\t\t\t\tw[l][j] = t;\n\t\t\t\t}\n\t\t\t}\n\t\t}\t\n\n\t\td = 1.0 / w[k][k];\n\t\tfor( i=(k+1); i <=(2); i++){\n\t\t\tif (w[i][k] == 0){\n\t\t\t\tcontinue;\n\t\t\t}\n\t\t\tt = w[i][k] * d;\n\t\t\tfor ( j = k; j <= (3); j++) {\n\t\t\t\tif (w[k][j] != 0){\n\t\t\t\t\tw[i][j] = w[i][j] - t * w[k][j];\n\t\t\t\t}\n\t\t\t}\n\t\t}\n\t}\n\tfor( i=(3); i >= 2; i--){\n\t\tfor( j=1; j <= i-1; j++){\n\t\t\tt = w[i - j - 1][i - 1]/w[ i -1][i - 1];\n\t\t\tw[i-j - 1][ 3] = w[i-j -1][3] - t*w[i - 1][ 3];\n\t\t}\n\t\tw[i-1][ 3] = w[i - 1][3]/w[ i -1][i - 1];\n\t}\n\tw[0][3] = w[0][3]/w[0][0];\n\tZn[0] = Z[0]+ w[0][3];\n\tZn[1] = Z[1]+ w[1][3];\n\tZn[2] = Z[2]+ w[2][3];\n\t\n\tdz = ( (Zn[0] - Z[0])**2 + (Zn[1] - Z[1])**2 + (Zn[2] - Z[2])**2 )**0.5;\n\tZ[0] = Zn[0];\n\tZ[1] = Zn[1];\n\tZ[2] = Zn[2];\n\n\tnnewt ++;\n}\n\nx[0] = Zn[0];\nx[1] = Zn[1];\nx[2] = Zn[2];"("x"=w98, "h"=w97, "b"=w96) -> ("x"=w99:dbl[])
      }
    }
    n17 = Not A Number/Path/Refnum?(number/path/refnum=w31) -> (NaN/Path/Refnum?=w34:bool)
    n18 = Greater Or Equal?(x=w31, y=w41) -> (x >= y?=w33:bool)
    n19 = Or(x=w34, y=w33) -> (x .or. y?=w32:bool)
    n20 = call "Extrapolator_Lorenz.vi"("Порядок экстраполятора"=2, "Dimension"=3, "Ext.Type"=w36, "Х - нач. условия"=w48, "n"=w44, "k"=w43) -> ("Tout"=w49:dbl[])  [unwired: 4 in, 1 out]
  }
  "Step Variation" <- w13
  "Number of steps" <- w23
  "Last Value" <- w11
  "Rejected Steps" <- w10
  "Last Value Reference" <- w4
  n21 = Compound Arithmetic op=ADD(invert w6, w5) -> (→"Real Error":dbl[][])
  n22 = case shown="4" "Error Analysis" {
    tunnel: w5 -> [w101 w109 w118 _ w129]
    tunnel: [w103 w111 w120 w127 w134] -> w8
    tunnel: w6 -> [w102 w110 w119 w126 w130]
    frame 1, Default {
      n23 = Compound Arithmetic op=ADD(invert w102, w101) -> (w100:dbl[][])
      n24 = for {
        tunnel: [w106] -> w104 mode=indexing
        tunnel: w100 -> [w105] mode=indexing
        n25 = call-poly <vilib>:"Vector Norm.vi"("Input Vector"=w105) -> ("norm"=w106:dbl)  [unwired: 9 in, 1 out]
      }
      n26 = Array Max & Min(array=w104) -> (max value=w103:dbl)  [unwired: 3 out]
    }
    frame 2 {
      n27 = Compound Arithmetic op=ADD(invert w110, w109) -> (w108:dbl[][])
      n28 = Transpose 2D Array(2D array=w108) -> (transposed array=w107:dbl[][])
      n29 = for {
        tunnel: [w114] -> w112 mode=indexing
        tunnel: w107 -> [w113] mode=indexing
        n30 = call-poly <vilib>:"Vector Norm.vi"("Input Vector"=w113) -> ("norm"=w114:dbl)  [unwired: 9 in, 1 out]
      }
      n31 = Array Max & Min(array=w112) -> (max value=w111:dbl)  [unwired: 3 out]
    }
    frame 3 {
      n32 = for {
        tunnel: w119 -> [w122] mode=indexing
        tunnel: [w122] -> w116
        tunnel: w118 -> [w121] mode=indexing
        tunnel: [w121] -> w117
      }
      n33 = Subtract(x=w117, y=w116) -> (x-y=w115:dbl[])
      n34 = call-poly <vilib>:"Vector Norm.vi"("Input Vector"=w115) -> ("norm"=w120:dbl)  [unwired: 9 in, 1 out]
    }
    frame 4 {
      n35 = for {
        tunnel: w126 -> [w128] mode=indexing
        tunnel: [w128] -> w125
      }
      n36 = Subtract(x="last_point_Thomas", y=w125) -> (x-y=w124:dbl[])
      n37 = call-poly <vilib>:"Vector Norm.vi"("Input Vector"=w124) -> ("norm"=w127:dbl)  [unwired: 9 in, 1 out]
    }
    frame 0 {
      n38 = Transpose 2D Array(2D array=w129) -> (transposed array=w132:dbl[][])
      n39 = Transpose 2D Array(2D array=w130) -> (transposed array=w133:dbl[][])
      n40 = Compound Arithmetic op=ADD(invert w133, w132) -> (w131:dbl[][])
      n41 = Absolute Value(x=w131) -> (abs(x)=w135:dbl[][])
      n42 = Array Max & Min(array=w135) -> (max value=w134:dbl)  [unwired: 3 out]
    }
  }
  "Error Estimation" <- w8
  n43 = Add Array Elements(numeric array=w10) -> (sum=→"Rejected steps":i32)
  n44 = Array Size(array=w13) -> (size(s)=w22:i32)
  n45 = for {
    N: "Points count" -> [_]
    tunnel: "k" -> [w159]
    tunnel: "n" -> [w158]
    tunnel: "Ext.Type" -> [w138]
    tunnel: "Initial Conditions" -> [w157]
    tunnel: w22 -> [w156]
    tunnel: [w149] -> w20 mode=indexing
    tunnel: "Шаг h, с" -> [w140]
    tunnel: "Hmin" -> [w148]
    tunnel: "Hmax" -> [w145]
    tunnel: "tolerance" -> [w144]
    tunnel: "Время, с" -> [w142]
    tunnel: "Parameter" -> [w136]
    n46 = flat-sequence {
      tunnel: w156 -> [w167]
      tunnel: w157 -> [w168]
      tunnel: w158 -> [w169]
      tunnel: w159 -> [w170]
      tunnel: [w170] -> w155
      tunnel: [w169] -> w154
      tunnel: [w168] -> w153
      tunnel: [w167] -> w152
      tunnel: [w166] -> w150
      tunnel: w148 -> [w165]
      tunnel: [w165] -> w147
      tunnel: w145 -> [w164]
      tunnel: [w164] -> w146
      tunnel: w144 -> [w163]
      tunnel: [w163] -> w143
      tunnel: w142 -> [w162]
      tunnel: [w162] -> w141
      tunnel: w140 -> [w161]
      tunnel: [w161] -> w139
      tunnel: w138 -> [w160]
      tunnel: [w160] -> w137
      tunnel: w155 -> [w182]
      tunnel: w154 -> [w181]
      tunnel: w153 -> [w180]
      tunnel: w152 -> [w179]
      tunnel: w147 -> [w177]
      tunnel: w146 -> [w176]
      tunnel: w143 -> [w175]
      tunnel: w141 -> [w174]
      tunnel: w139 -> [w173]
      tunnel: w137 -> [w172]
      tunnel: w136 -> [w171]
      tunnel: [w229] -> w151
      frame #0 {
        n47 = call <vilib>:"High Resolution Relative Seconds.vi"() -> ("relative seconds"=w166:dbl)
      }
      frame #1 {
        n48 = for {
          N: w179 -> [_]
          shift-right: [w192] -> _
          shift-left: w180 -> [w194]
          tunnel: w181 -> [w196]
          tunnel: w182 -> [w191]
          tunnel: w172 -> [w195]
          shift-right: [w193] -> _
          shift-left: w173 -> [w186]
          tunnel: w177 -> [w190]
          tunnel: w176 -> [w189]
          tunnel: w175 -> [w188]
          shift-right: [w185] -> _
          shift-left: 0.0 -> [w184]
          tunnel: w174 -> [w187]
          tunnel: w171 -> [w183]
          n49 = while {
            tunnel: w196 -> [w206]
            tunnel: w195 -> [w221]
            tunnel: w194 -> [w204]
            tunnel: [w199] -> w192
            tunnel: w191 -> [w205]
            tunnel: w190 -> [w217]
            tunnel: w189 -> [w216]
            tunnel: w188 -> [w215]
            tunnel: w184 -> [w214]
            tunnel: w187 -> [w213]
            shift-right: [w218] -> w193
            shift-left: w186 -> [w203]
            tunnel: [w207] -> w185
            tunnel: w183 -> [w201]
            i -> [w209]
            stop <- w210 stop-if-true
            n50 = for {
              N: w205 -> [_]
              tunnel: w206 -> [w227] mode=indexing
              tunnel: w203 -> [w228]
              tunnel: w204 -> [w224]
              tunnel: [w223] -> w202 mode=indexing
              tunnel: w201 -> [w222]
              n51 = Compound Arithmetic op=MULTIPLY(w228, invert w227) -> (w225:dbl)
              n52 = Decrement(x=w227) -> (x-1=w226:i32)
              n53 = formula code="int i;\n//cromer 1\nx1[0]=x[0]+h*(-b[0]*x[0]-4*(x[1]+x[2])-x[1]*x[1]);\nx1[1]=x[1]+h*(-b[1]*x[1]-4*(x[0]+x[2])-x[2]*x[2]);\nx1[2]=x[2]+h*(-b[2]*x[2]-4*(x[1]+x[0])-x[0]*x[0]);\n\nh=2*h;\nfor (i = 0; i<N; i++)\n{\n//EEuler\nx2[0]=x[0]+h*(-b[0]*x1[0]-4*(x1[1]+x1[2])-x1[1]*x1[1]);\nx2[1]=x[1]+h*(-b[1]*x1[1]-4*(x1[0]+x1[2])-x1[2]*x1[2]);\nx2[2]=x[2]+h*(-b[2]*x1[2]-4*(x1[1]+x1[0])-x1[0]*x1[0]);\n\nx[0]=x1[0];\nx[1]=x1[1];\nx[2]=x1[2];\nx1[0]=x2[0];\nx1[1]=x2[1];\nx1[2]=x2[2];\n};\n\nh=h*0.5;\nx2[0]=(x[0]+x1[0]+h*(-b[0]*x1[0]-4*(x1[1]+x1[2])-x1[1]*x1[1]))/2;\nx2[1]=(x[1]+x1[1]+h*(-b[1]*x1[1]-4*(x1[0]+x1[2])-x1[2]*x1[2]))/2;\nx2[2]=(x[2]+x1[2]+h*(-b[2]*x1[2]-4*(x1[1]+x1[0])-x1[0]*x1[0]))/2;"("x"=w224, "x1"=w224, "h"=w225, "x2"=w224, "N"=w226, "b"=w222) -> ("x2"=w223:dbl[])
            }
            n54 = call "Extrapolator_Lorenz.vi"("Порядок экстраполятора"=2 ("input variable"), "Dimension"=3 ("input variable"), "Ext.Type"=w221, "Х - нач. условия"=w202, "n"=w206, "k"=w205) -> ("TPrev"=w198:dbl[], "Tout"=w199:dbl[])  [unwired: 4 in]
            n55 = Subtract(x=w199, y=w198) -> (x-y=w200:dbl[])
            n56 = Equal?(x=w209, y=10) -> (x = y?=w211:bool)
            n57 = call-poly <vilib>:"Vector Norm.vi"("Input Vector"=w200) -> ("norm"=w197:dbl)  [unwired: 9 in, 1 out]
            n58 = call "Common_StepVariator.vi"("err"=w197, "tolerance"=w215, "Hmax"=w216, "Шаг h, с"=w203, "Current time"=w214, "k"=w205, "Hmin"=w217, "tmax"=w213) -> ("Hnew"=w218:dbl, "New time"=w207:dbl, "stop"=w208:bool)  [unwired: 4 in, 1 out]
            n59 = Or(x=w211, y=w208) -> (x .or. y?=w210:bool)
          }
        }
      }
      frame #2 {
        n60 = call <vilib>:"High Resolution Relative Seconds.vi"() -> ("relative seconds"=w229:dbl)
      }
    }
    n61 = Subtract(x=w151, y=w150) -> (x-y=w149:dbl)
  }
  "Step time variation" <- w20
  n62 = case shown="True" TRUE {
    tunnel: w20 -> [w230 w233]
    tunnel: [w231 w232] -> w19
    frame False {
      n63 = call-poly <vilib>:"RMS.vi"("X"=w230) -> ("rms value"=w231:dbl)  [unwired: 1 out]
    }
    frame True {
      n64 = call <vilib>:"Median.vi"("X"=w233) -> ("median"=w232:dbl)  [unwired: 1 out]
    }
  }
  "Elapsed Time" <- w19
